vi "Array Edit.vi"(9 "Number of Points":dbl, 11 "Y-values":dbl[](array[numeric])) -> (3 "Editted Y Values":dbl[](array[numeric]))   [LabVIEW 2014]
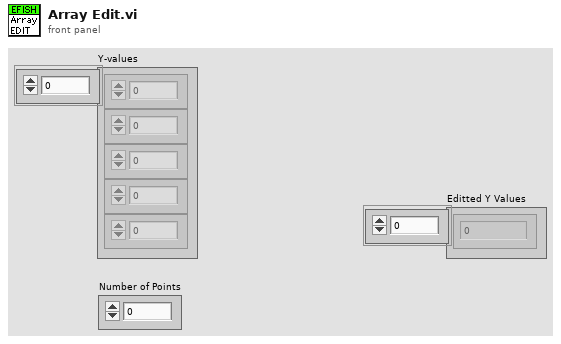
[diagram p1: front panel]
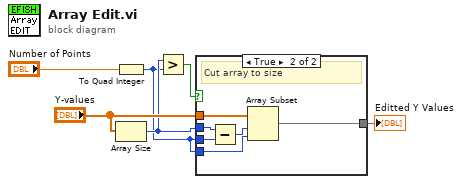
[diagram p0: block diagram]
diagram:
  n1 = To Quad Integer(1:"Number of Points") -> (0:w2:i64)
  n2 = Array Size(array="Y-values") -> (size(s)=w3:i32)
  n3 = Greater?(x=w3, y=w2) -> (0:w5:bool)
  n4 = case shown="True" w5 {
    tunnel: "Y-values" -> [w7 w13]
    tunnel: w2 -> [_ w12]
    tunnel: w3 -> [_ w11]
    tunnel: w2 -> [_ w10]
    tunnel: [w7 w8] -> w1
    frame False {
      # "no need to edit"
    }
    frame True {
      # "Cut array to size"
      n5 = Subtract(x=w11, y=w10) -> (x-y=w9:i64)
      n6 = Array Subset(array=w13, index=w9, length=w12) -> (w8:dbl[])
    }
  }
  "Editted Y Values" <- w1
